vi "AlazarConfigureAuxIO.vi"(3 "error in (no error)":errorcluster, 4 "Parameter":u32, 5 "Mode":u32, 6 "Handle":u64) -> (0 "error out":errorcluster, 1 "Return Code":u32, 2 "Handle":u64)   [LabVIEW 2018]
doc: "Configure the AUX I/O connector as an input or output signal."
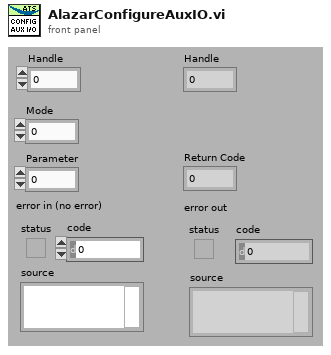
[diagram p1: front panel]
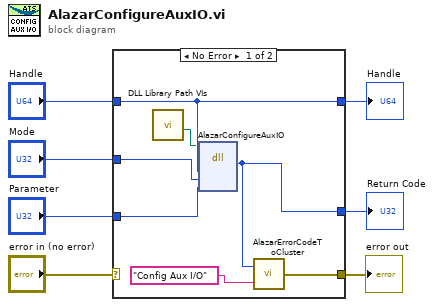
[diagram p0: block diagram]
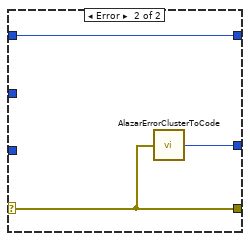
[diagram p2: hidden frame]
diagram:
  n1 = case shown="No Error" "error in (no error)" {
    selector: "error in (no error)" -> [_ w17]
    tunnel: [w10 w17] -> w6
    tunnel: [w11 w16] -> w5
    tunnel: "Handle" -> [w12 w15]
    tunnel: [w12 w15] -> w3
    tunnel: "Mode" -> [w14 _]
    tunnel: "Parameter" -> [w13 _]
    frame No Error {
      n2 = call "DLL Library Path VIs.vi"() -> ("Alazar"=w8:path)  [unwired: 5 in, 6 out]
      n3 = dll-call lib="C:/Project/SerialSectOCT - FFT GPU/SerialSectOCT/Labview Software/DLL/ATSApi.dll" fn="AlazarConfigureAuxIO"(path in=w8, "handle"=w12, "mode"=w14, "parameter"=w13) -> ("return type"=w11:u32)  [unwired: 5 in, 2 out]
      n4 = call "AlazarErrorCodeToCluster.vi"("Message"="Config Aux I/O", "Error Code"=w11) -> ("error out"=w10:errorcluster)
    }
    frame Error {
      n5 = call "AlazarErrorClusterToCode.vi"("error in (no error)"=w17) -> ("Error Code"=w16:u32)
    }
  }
  "Handle" <- w3
  "error out" <- w6
  "Return Code" <- w5
